vi "SaveWaveformsASCII.vi"(4 "transpose? (yes:T)":bool=TRUE, 5 "format":string="%.6g", 6 "Deafault channel name prefix":string="CH", 7 "Channel name attribute":string="NI_ChannelName", 8 "error in":errorcluster, 9 "Save column names":bool, 10 "waveforms in":waveform(dbl)[](array[waveform]), 11 "file (use dialog)":path) -> (0 "error out":errorcluster)   [LabVIEW 2015]
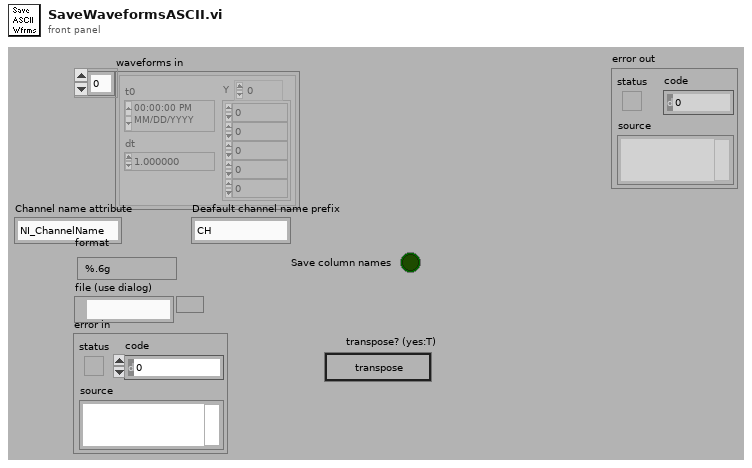
[diagram p1: front panel]
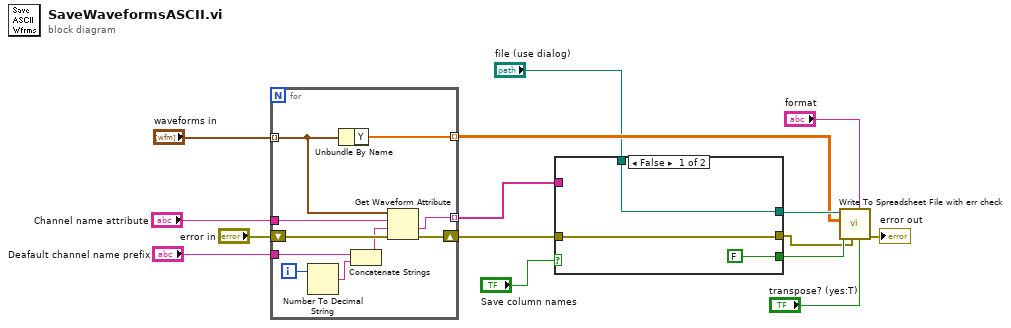
[diagram p0: block diagram]
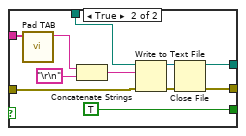
[diagram p2: hidden frame]
diagram:
  n1 = for {
    tunnel: "waveforms in" -> [w24] mode=indexing
    tunnel: [w25] -> w10 mode=indexing
    tunnel: "Channel name attribute" -> [w23]
    tunnel: "Deafault channel name prefix" -> [w22]
    shift-right: [w20] -> w6
    shift-left: "error in" -> [w21]
    tunnel: [w16] -> w7 mode=indexing
    i -> [w18]
    n2 = Number To Decimal String(number=w18) -> (decimal integer string=w17:string)  [unwired: 1 out]
    n3 = Unbundle By Name(w24) -> ("Y"=w25:dbl[])
    n4 = Concatenate Strings(w22, w17) -> (w19:string)
    n5 = Get Waveform Attribute(4:w21, 5:w19, 6:w23, 7:w24) -> (0:w20:errorcluster, 1:w16:string)  [unwired: 2 out]
  }
  n6 = case shown="False" "Save column names" {
    tunnel: [FALSE ("append to file? (new file:F)") TRUE] -> w14
    tunnel: [w26 w33] -> w13
    tunnel: w7 -> [_ w37]
    tunnel: [w27 w31] -> w12
    tunnel: w6 -> [w26 w30]
    tunnel: "file (use dialog)" -> [w27 w29]
    frame False {
    }
    frame True {
      n7 = call "Pad TAB.vi"("Input String Array"=w37) -> ("Output String"=w38:string)  [unwired: 1 in, 9 out]
      n8 = Concatenate Strings(w38, "\r\n") -> (w36:string)
      n9 = Write to Text File(file (use dialog)=w29, text=w36, error in=w30) -> (refnum out=w32:refnum<file>, error out=w34:errorcluster)  [unwired: 2 out]
      n10 = Close File(refnum=w32, error in=w34) -> (path=w31:path, error out=w33:errorcluster)
    }
  }
  n11 = call "Write To Spreadsheet File with err check.vi"("transpose? (no:F)"="transpose? (yes:T)", "format (%.3f)"="format", "error in (no error)"=w13, "append to file? (new file:F)"=w14, "2D data"=w10, "file path (dialog if empty)"=w12) -> ("error out"=→"error out":errorcluster)  [unwired: 2 in, 3 out]
